vi "Interpret Driver Controls.vi"() -> ()   [LabVIEW 2018]
uses:
  <vilib>/Rock Robotics/WPI/DriverStation/WPI_DriverStationDerivedRobotMode.ctl
  Robot Global Data.vi
  SubSystems/Controllers/Driver Controller/Driver Controller Global.vi
  SubSystems/Lift/Lift Global.vi
  SubSystems/Drive Train/Drive Train Global.vi
  SubSystems/Controllers/Manipulator Controlller/Manipulator Controller Global.vi
  SubSystems/HAB Climber/HAB Climber Global.vi
  SubSystems/Cargo Intake/Cargo Intake Global.vi
  SubSystems/Hatch Panel Intake/Hatch Panel Intake Global.vi
  <vilib>/addons/control/pid/pid.llb/PID (DBL).vi
  <vilib>/addons/control/pid/NI_PID_pid.lvlib
panel:
  in  "Rot. Point Y":dbl
  in  "Rot. Point X":dbl
  in  "robot centric":bool
  in  "Z speed":dbl=1.0
  in  "Y Speed":dbl=1.0
  in  "X Speed":dbl=1.0
  out "Grab Hatch Boolean Thing":bool=TRUE
  in  "Track Scale":dbl
  in  "Last Move Deadband":u32=500
  in  "Last Time Auto":u32=1816077
  in  "Camera Tracking":T1={"proportional gain (Kc)"=0.06, "integral time (Ti, min)"=0.0, "derivative time (Td, min)"=0.0}
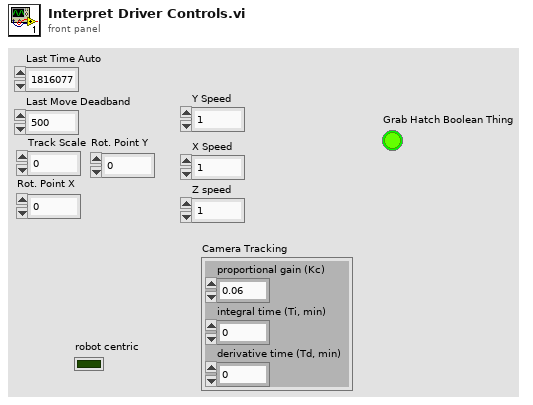
[diagram p1: front panel]
types:
  T1 = cluster{"proportional gain (Kc)":dbl, "integral time (Ti, min)":dbl, "derivative time (Td, min)":dbl}
  T2 = enum16{"Manual", "Hatch Panel Zone 1", "Hatch Panel Zone 2", "Hatch Panel Zone 3", "Cargo Zone 1", "Cargo Zone 2", "Cargo Zone 3", "Cargo Ship Zone"}
  T3 = enum16{"Hatch Panel Zone 1", "Hatch Panel Zone 2", "Hatch Panel Zone 3", "Cargo Zone 1", "Cargo Zone 2", "Cargo Zone 3", "Cargo Ship Zone"}
  T4 = typedef "WPI_DriverStationDerivedRobotMode.ctl" = enum16{"Init", "Execute", "Stop"}
  T5 = cluster{"Rollover":dbl, "Yaw":dbl, "Cont Yaw":dbl}
  T6 = cluster{"offsetAngle H":dbl, "offsetAngle V":dbl, "area":dbl, "skew":dbl, "validTarget":dbl, "latency":dbl}
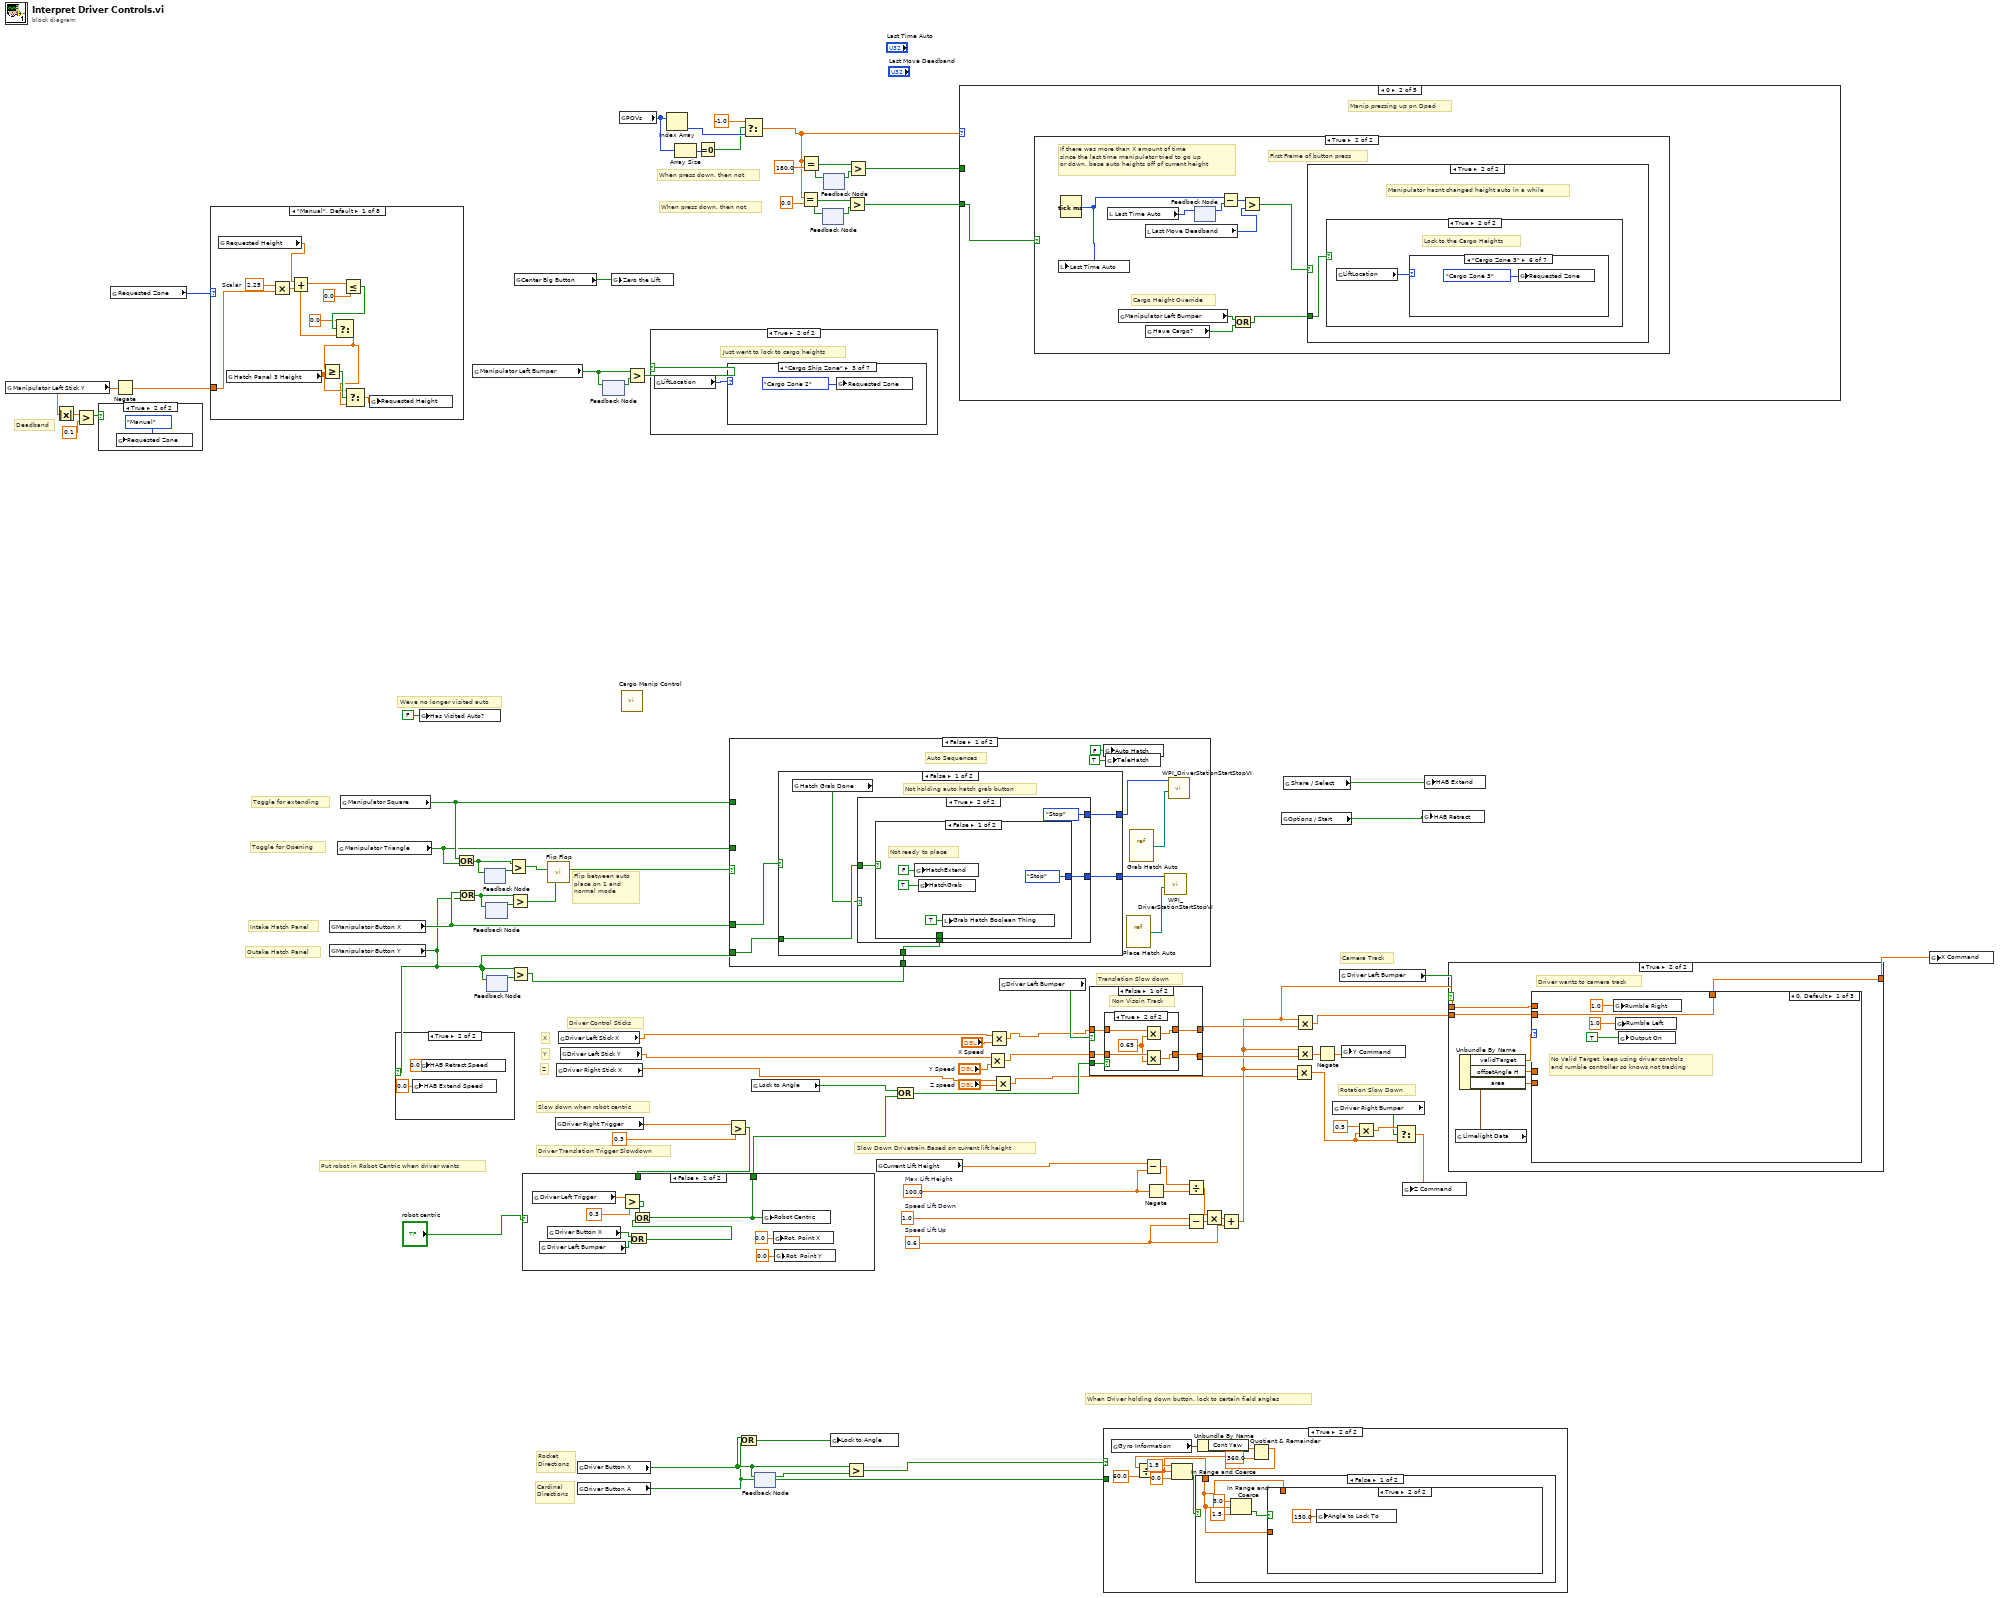
[diagram p0: block diagram]
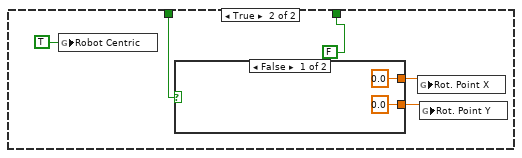
[diagram p3: hidden frame]
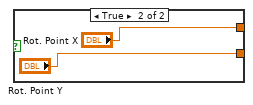
[diagram p4: hidden frame]
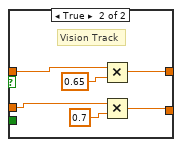
[diagram p6: hidden frame]
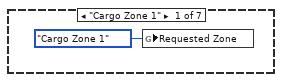
[diagram p8: hidden frame]
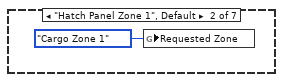
[diagram p9: hidden frame]
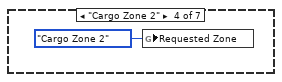
[diagram p10: hidden frame]
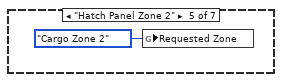
[diagram p11: hidden frame]
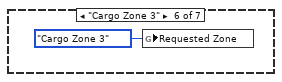
[diagram p12: hidden frame]
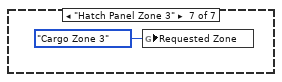
[diagram p13: hidden frame]
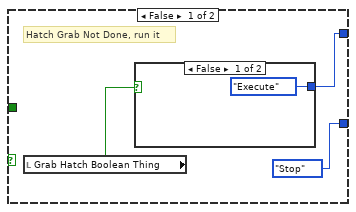
[diagram p14: hidden frame]
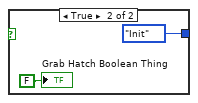
[diagram p15: hidden frame]
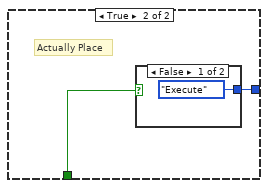
[diagram p16: hidden frame]
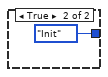
[diagram p17: hidden frame]
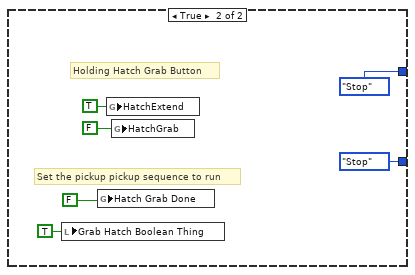
[diagram p18: hidden frame]
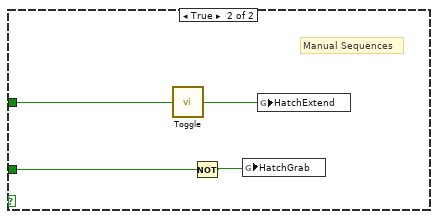
[diagram p19: hidden frame]
diagram:
  w70 = 0.6  # Speed Lift Up
  w74 = 1.0  # Speed Lift Down
  w68 = 100.0  # Max Lift Height
  # "Toggle for Opening"
  # "Toggle for extending"
  # "Outake Hatch Panel"
  # "Intake Hatch Panel"
  # "Flip between auto\nplace on 1 and \nnormal mode"
  # "When press down, then not"
  # "When press down, then not"
  # "Deadband"
  # "Weve no longer visited auto"
  # "Camera Track"
  # "Rotation Slow Down"
  # "Rocket\nDirections"
  # "Cardinal\nDirections"
  # "When Driver holding down button, lock to certain field angles"
  # "Slow Down Drivetrain Based on current lift height"
  # "Put robot in Robot Centric when driver wants"
  # "Slow down when robot centric"
  # "Driver Translation Trigger Slowdown"
  # "Translation Slow down"
  # "Z"
  # "Y"
  # "X"
  # "Driver Control Sticks"
  n1 = global read "Manipulator Controller Global.vi" "Manipulator Left Stick Y"() -> (w44:dbl)
  n2 = Absolute Value(x=w44) -> (abs(x)=w47:dbl)
  n3 = Greater?(x=w47, y=0.1) -> (0:w45:bool)
  n4 = case shown="True" w45 {
    frame False {
    }
    frame True {
      n5 = global write "Lift Global.vi" "Requested Zone"(T2."Manual" ("Requested Zone")) -> ()
    }
  }
  n6 = global read "Lift Global.vi" "Requested Zone"() -> (w48:T2)
  n7 = Negate(x=w44) -> (-x=w43:dbl)
  n8 = case shown="\"Manual\", Default" w48 {
    tunnel: w43 -> [w95 _ _ _ _ _ _ _]
    frame "Manual", Default {
      w94 = 2.25  # Scalar
      n9 = global read "Lift Global.vi" "Requested Height"() -> (w97:dbl)
      n10 = global read "Lift Global.vi" "Hatch Panel 3 Height"() -> (w88:dbl)
      n11 = Multiply(x=w94, y=w95) -> (x*y=w96:dbl)
      n12 = Add(x=w97, y=w96) -> (x+y=w90:dbl)
      n13 = Less Or Equal?(x=w90, y=0.0) -> (x <= y?=w92:bool)
      n14 = Select(t=0.0, s=w92, f=w90) -> (s? t:f=w87:dbl)
      n15 = Greater Or Equal?(x=w87, y=w88) -> (x >= y?=w89:bool)
      n16 = Select(t=w88, s=w89, f=w87) -> (s? t:f=w86:dbl)
      n17 = global write "Lift Global.vi" "Requested Height"(w86) -> ()
    }
    frame "Hatch Panel Zone 1" {
      n18 = global read "Lift Global.vi" "Hatch Panel 1 Height"() -> (w98:dbl)
      n19 = global write "Lift Global.vi" "Requested Height"(w98) -> ()
    }
    frame "Hatch Panel Zone 2" {
      n20 = global read "Lift Global.vi" "Hatch Panel 2 Height"() -> (w99:dbl)
      n21 = global write "Lift Global.vi" "Requested Height"(w99) -> ()
    }
    frame "Hatch Panel Zone 3" {
      n22 = global read "Lift Global.vi" "Hatch Panel 3 Height"() -> (w100:dbl)
      n23 = global write "Lift Global.vi" "Requested Height"(w100) -> ()
    }
    frame "Cargo Zone 1" {
      n24 = global read "Lift Global.vi" "Cargo Zone 1 Height"() -> (w101:dbl)
      n25 = global write "Lift Global.vi" "Requested Height"(w101) -> ()
    }
    frame "Cargo Zone 2" {
      n26 = global read "Lift Global.vi" "Cargo Zone 2 Height"() -> (w102:dbl)
      n27 = global write "Lift Global.vi" "Requested Height"(w102) -> ()
    }
    frame "Cargo Zone 3" {
      n28 = global read "Lift Global.vi" "Cargo Zone 3 Height"() -> (w103:dbl)
      n29 = global write "Lift Global.vi" "Requested Height"(w103) -> ()
    }
    frame "Cargo Ship Zone" {
      n30 = global read "Lift Global.vi" "Cargo Ship Height"() -> (w104:dbl)
      n31 = global write "Lift Global.vi" "Requested Height"(w104) -> ()
    }
  }
  n32 = global read "Manipulator Controller Global.vi" "Manipulator Button X"() -> (w20:bool)
  n33 = global read "Manipulator Controller Global.vi" "Manipulator Button Y"() -> (w4:bool)
  n34 = global read "Manipulator Controller Global.vi" "Manipulator Triangle"() -> (w30:bool)
  n35 = global read "Manipulator Controller Global.vi" "Manipulator Square"() -> (w31:bool)
  n36 = case shown="True" w4 {
    frame False {
    }
    frame True {
      n37 = global write "HAB Climber Global.vi" "HAB Extend Speed"(0.0 ("HAB Extend Speed")) -> ()
      n38 = global write "HAB Climber Global.vi" "HAB Retract Speed"(0.0 ("HAB Retract Speed")) -> ()
    }
  }
  n39 = global write "Robot Global Data.vi" "Has Visited Auto?"(FALSE ("Has Visited Auto?")) -> ()
  n40 = Or(x=w31, y=w30) -> (x .or. y?=w28:bool)
  n41 = Or(x=w20, y=w4) -> (x .or. y?=w25:bool)
  n42 = global read "Manipulator Controller Global.vi" "Manipulator Left Bumper"() -> (w18:bool)
  n43 = feedback-in #1(w28) -> ()
  n44 = feedback #1() -> (w29:bool)  [unwired: 1 in]
  n45 = feedback #2() -> (w26:bool)  [unwired: 1 in]
  n46 = feedback-in #2(w25) -> ()
  n47 = feedback #3() -> (w22:bool)  [unwired: 1 in]
  n48 = feedback-in #3(w4) -> ()
  n49 = Greater?(x=w28, y=w29) -> (0:w27:bool)
  n50 = Greater?(x=w25, y=w26) -> (0:w24:bool)
  n51 = Greater?(x=w4, y=w22) -> (0:w21:bool)
  n52 = global read "Manipulator Controller Global.vi" "Center Big Button"() -> (w14:bool)
  n53 = call "Flip Flop.vi"("Line 2"=w24, "Line 1"=w27) -> ("Switch"=w23:bool)  [unwired: 9 in]
  n54 = global read "Driver Controller Global.vi" "Driver Right Trigger"() -> (w84:dbl)
  n55 = global read "Driver Controller Global.vi" "Driver Right Stick X"() -> (w7:dbl)
  n56 = global read "Driver Controller Global.vi" "Driver Left Stick X"() -> (w16:dbl)
  n57 = global read "Driver Controller Global.vi" "Driver Left Stick Y"() -> (w15:dbl)
  n58 = global read "Driver Controller Global.vi" "Driver Button X"() -> (w66:bool)
  n59 = global read "Driver Controller Global.vi" "Driver Button A"() -> (w64:bool)
  n60 = feedback #4() -> (w19:bool)  [unwired: 1 in]
  n61 = feedback-in #4(w18) -> ()
  n62 = global write "Lift Global.vi" "Zero the Lift"(w14) -> ()
  n63 = global read "Manipulator Controller Global.vi" "POVs"() -> (w52:i16[])
  n64 = call "Cargo Manip Control.vi"() -> ()  [unwired: 12 in]
  n65 = Greater?(x=w18, y=w19) -> (0:w17:bool)
  n66 = case shown="True" w17 {
    frame False {
    }
    frame True {
      # "Just went to lock to cargo heights"
      n67 = global read "Lift Global.vi" "LiftLocation"() -> (w107:T3)
      n68 = case shown="\"Cargo Ship Zone\"" w107 {
        frame "Cargo Zone 1" {
          n69 = global write "Lift Global.vi" "Requested Zone"(T2."Cargo Zone 1" ("Requested Zone")) -> ()
        }
        frame "Hatch Panel Zone 1", Default {
          n70 = global write "Lift Global.vi" "Requested Zone"(T2."Cargo Zone 1" ("Requested Zone")) -> ()
        }
        frame "Cargo Ship Zone" {
          n71 = global write "Lift Global.vi" "Requested Zone"(T2."Cargo Zone 2" ("Requested Zone")) -> ()
        }
        frame "Cargo Zone 2" {
          n72 = global write "Lift Global.vi" "Requested Zone"(T2."Cargo Zone 2" ("Requested Zone")) -> ()
        }
        frame "Hatch Panel Zone 2" {
          n73 = global write "Lift Global.vi" "Requested Zone"(T2."Cargo Zone 2" ("Requested Zone")) -> ()
        }
        frame "Cargo Zone 3" {
          n74 = global write "Lift Global.vi" "Requested Zone"(T2."Cargo Zone 3" ("Requested Zone")) -> ()
        }
        frame "Hatch Panel Zone 3" {
          n75 = global write "Lift Global.vi" "Requested Zone"(T2."Cargo Zone 3" ("Requested Zone")) -> ()
        }
      }
    }
  }
  n76 = Index Array(array=w52) -> (element=w49:i16)  [unwired: 1 in]
  n77 = Array Size(array=w52) -> (size(s)=w51:i32)
  n78 = Equal To 0?(x=w51) -> (x = 0?=w42:bool)
  n79 = Greater?(x=w84, y=0.3) -> (0:w5:bool)
  n80 = case shown="False" "robot centric" {
    tunnel: [w117 FALSE] -> w12
    tunnel: w5 -> [_ w126]
    frame False {
      n81 = global read "Driver Controller Global.vi" "Driver Left Trigger"() -> (w122:dbl)
      n82 = global read "Driver Controller Global.vi" "Driver Left Bumper"() -> (w118:bool)
      n83 = global read "Driver Controller Global.vi" "Driver Button X"() -> (w119:bool)
      n84 = Greater?(x=w122, y=0.3) -> (0:w121:bool)
      n85 = Or(x=w119, y=w118) -> (x .or. y?=w120:bool)
      n86 = Or(x=w121, y=w120) -> (x .or. y?=w117:bool)
      n87 = global write "Drive Train Global.vi" "Robot Centric"(w117) -> ()
      n88 = global write "Drive Train Global.vi" "Rot. Point X"(0.0 ("Rot. Point X")) -> ()
      n89 = global write "Drive Train Global.vi" "Rot. Point Y"(0.0 ("Rot. Point Y")) -> ()
    }
    frame True {
      n90 = global write "Drive Train Global.vi" "Robot Centric"(TRUE ("Robot Centric")) -> ()
      n91 = case shown="False" w126 {
        tunnel: [0.0 ("Rot. Point Y") "Rot. Point Y"] -> w125
        tunnel: [0.0 ("Rot. Point X") "Rot. Point X"] -> w124
        frame False {
        }
        frame True {
        }
      }
      n92 = global write "Drive Train Global.vi" "Rot. Point X"(w124) -> ()
      n93 = global write "Drive Train Global.vi" "Rot. Point Y"(w125) -> ()
    }
  }
  n94 = case shown="False" w23 {
    tunnel: w30 -> [_ w172]
    tunnel: w31 -> [_ w173]
    tunnel: w20 -> [w141 _]
    tunnel: w21 -> [w138 _]
    tunnel: w4 -> [w137 _]
    frame False {
      # "Auto Sequences"
      n95 = case shown="False" w141 {
        tunnel: [w146 WPI_DriverStationDerivedRobotMode."Stop" ("Call Context")] -> w139
        tunnel: w138 -> [w145 _]
        tunnel: w137 -> [w144 _]
        tunnel: [w142 WPI_DriverStationDerivedRobotMode."Stop" ("Call Context")] -> w135
        frame False {
          # "Not holding auto hatch grab button"
          n96 = global read "Hatch Panel Intake Global.vi" "Hatch Grab Done"() -> (w143:bool)
          n97 = case shown="True" w143 {
            tunnel: [WPI_DriverStationDerivedRobotMode."Stop" ("Call Context") w156] -> w146
            tunnel: w145 -> [_ w155]
            tunnel: w144 -> [_ w154]
            tunnel: [w149 WPI_DriverStationDerivedRobotMode."Stop" ("Call Context")] -> w142
            frame False {
              # "Hatch Grab Not Done, run it"
              n98 = local read "Grab Hatch Boolean Thing"() -> (w147:bool)
              n99 = case shown="False" w147 {
                tunnel: [WPI_DriverStationDerivedRobotMode."Execute" ("Call Context") WPI_DriverStationDerivedRobotMode."Init" ("Call Context")] -> w149
                frame False {
                }
                frame True {
                  "Grab Hatch Boolean Thing" <- FALSE ("Grab Hatch Boolean Thing")
                }
              }
            }
            frame True {
              n100 = case shown="False" w154 {
                tunnel: [WPI_DriverStationDerivedRobotMode."Stop" ("Call Context") w162] -> w156
                tunnel: w155 -> [_ w161]
                frame False {
                  # "Not ready to place"
                  n101 = global write "Hatch Panel Intake Global.vi" "HatchExtend"(FALSE ("HatchExtend")) -> ()
                  n102 = global write "Hatch Panel Intake Global.vi" "HatchGrab"(TRUE ("HatchExtend")) -> ()
                  n103 = local write "Grab Hatch Boolean Thing"(TRUE ("Grab Hatch Boolean Thing")) -> ()
                }
                frame True {
                  # "Actually Place"
                  n104 = case shown="False" w161 {
                    tunnel: [WPI_DriverStationDerivedRobotMode."Execute" ("Call Context") WPI_DriverStationDerivedRobotMode."Init" ("Call Context")] -> w162
                    frame False {
                    }
                    frame True {
                    }
                  }
                }
              }
            }
          }
        }
        frame True {
          # "Set the pickup pickup sequence to run"
          # "Holding Hatch Grab Button"
          n105 = local write "Grab Hatch Boolean Thing"(TRUE ("Grab Hatch Boolean Thing")) -> ()
          n106 = global write "Hatch Panel Intake Global.vi" "Hatch Grab Done"(FALSE ("HatchExtend")) -> ()
          n107 = global write "Hatch Panel Intake Global.vi" "HatchExtend"(TRUE ("HatchExtend")) -> ()
          n108 = global write "Hatch Panel Intake Global.vi" "HatchGrab"(FALSE ("HatchExtend")) -> ()
        }
      }
      n109 = global write "Hatch Panel Intake Global.vi" "Auto Hatch"(FALSE ("TeleHatch")) -> ()
      n110 = global write "Hatch Panel Intake Global.vi" "TeleHatch"(TRUE ("TeleHatch")) -> ()
      n111 = vi-ref "Place Hatch Auto.vi"() -> (w140:refnum<vi>)
      n112 = vi-ref "Grab Hatch Auto.vi"() -> (w136:refnum<vi>)
      n113 = call <vilib>:"WPI_DriverStationStartStopVI.vi"("VI in"=w140, "Call Context"=w139) -> ()  [unwired: 10 in]
      n114 = call <vilib>:"WPI_DriverStationStartStopVI.vi"("VI in"=w136, "Call Context"=w135) -> ()  [unwired: 10 in]
    }
    frame True {
      # "Manual Sequences"
      n115 = call "Toggle.vi"("Input"=w173) -> ("Output"=w174:bool)
      n116 = Not(x=w172) -> (.not. x?=w171:bool)
      n117 = global write "Hatch Panel Intake Global.vi" "HatchGrab"(w171) -> ()
      n118 = global write "Hatch Panel Intake Global.vi" "HatchExtend"(w174) -> ()
    }
  }
  n119 = Or(x=w66, y=w64) -> (x .or. y?=w63:bool)
  n120 = Select(t=-1.0, s=w42, f=w49) -> (s? t:f=w34:dbl)
  n121 = global read "Drive Train Global.vi" "Lock to Angle"() -> (w62:bool)
  n122 = feedback #5() -> (w67:bool)  [unwired: 1 in]
  n123 = feedback-in #5(w66) -> ()
  n124 = Equal?(x=w34, y=0.0) -> (x = y?=w37:bool)
  n125 = Equal?(x=w34, y=180.0) -> (x = y?=w39:bool)
  n126 = feedback #6() -> (w36:bool)  [unwired: 1 in]
  n127 = feedback-in #6(w37) -> ()
  n128 = feedback-in #7(w39) -> ()
  n129 = feedback #7() -> (w40:bool)  [unwired: 1 in]
  n130 = global write "Drive Train Global.vi" "Lock to Angle"(w63) -> ()
  n131 = Greater?(x=w66, y=w67) -> (0:w65:bool)
  n132 = Greater?(x=w37, y=w36) -> (0:w33:bool)
  n133 = Greater?(x=w39, y=w40) -> (0:w38:bool)
  n134 = global read "Lift Global.vi" "Current Lift Height"() -> (w76:dbl)
  n135 = Compound Arithmetic op=OR(w62, w12) -> (w9:bool)
  n136 = case shown="0" w34 {
    tunnel: w38 -> [_ _ w219 _ _]
    tunnel: w33 -> [_ w175 _ _ _]
    frame -1, Default {
      # "Nothing on the D-Pad is pressed!"
    }
    frame 0 {
      # "Manip pressing up on Dpad"
      n137 = case shown="True" w175 {
        frame False {
          # "Still pressing button, do nothing"
        }
        frame True {
          # "Cargo Height Override"
          # "First Frame of button press"
          # "If there was more than X amount of time\nsince the last time manipulator tried to go up\nor down, base auto heights off of current height"
          n138 = Tick Count (ms)() -> (millisecond timer value=w181:u32)
          n139 = local write "Last Time Auto"(w181) -> ()
          n140 = local read "Last Time Auto"() -> (w180:u32)
          n141 = global read "Manipulator Controller Global.vi" "Manipulator Left Bumper"() -> (w178:bool)
          n142 = local read "Last Move Deadband"() -> (w182:u32)
          n143 = global read "Cargo Intake Global.vi" "Have Cargo?"() -> (w176:bool)
          n144 = feedback #8() -> (w179:u32)  [unwired: 1 in]
          n145 = feedback-in #8(w180) -> ()
          n146 = Subtract(x=w181, y=w179) -> (x-y=w184:u32)
          n147 = Or(x=w178, y=w176) -> (x .or. y?=w177:bool)
          n148 = Greater?(x=w184, y=w182) -> (0:w183:bool)
          n149 = case shown="True" w183 {
            tunnel: w177 -> [w185 w202]
            frame False {
              # "Manipulator is still changing height to go to"
              n150 = case shown="False" w185 {
                frame False {
                  # "Lock to the Hatch Heights"
                  n151 = global read "Lift Global.vi" "Requested Zone"() -> (w186:T2)
                  n152 = case shown="\"Hatch Panel Zone 3\"" w186 {
                    frame "Manual" {
                    }
                    frame "Cargo Zone 1" {
                      n153 = global write "Lift Global.vi" "Requested Zone"(T2."Hatch Panel Zone 1" ("Requested Zone")) -> ()
                    }
                    frame "Hatch Panel Zone 1", Default {
                      n154 = global write "Lift Global.vi" "Requested Zone"(T2."Hatch Panel Zone 2" ("Requested Zone")) -> ()
                    }
                    frame "Cargo Ship Zone" {
                      n155 = global write "Lift Global.vi" "Requested Zone"(T2."Hatch Panel Zone 2" ("Requested Zone")) -> ()
                    }
                    frame "Cargo Zone 2" {
                      n156 = global write "Lift Global.vi" "Requested Zone"(T2."Hatch Panel Zone 2" ("Requested Zone")) -> ()
                    }
                    frame "Hatch Panel Zone 2" {
                      n157 = global write "Lift Global.vi" "Requested Zone"(T2."Hatch Panel Zone 3" ("Requested Zone")) -> ()
                    }
                    frame "Cargo Zone 3" {
                      n158 = global write "Lift Global.vi" "Requested Zone"(T2."Hatch Panel Zone 3" ("Requested Zone")) -> ()
                    }
                    frame "Hatch Panel Zone 3" {
                      n159 = global write "Lift Global.vi" "Requested Zone"(T2."Hatch Panel Zone 3" ("Requested Zone")) -> ()
                    }
                  }
                }
                frame True {
                  # "Lock to the Cargo Heights"
                  n160 = global read "Lift Global.vi" "Requested Zone"() -> (w194:T2)
                  n161 = case shown="\"Manual\"" w194 {
                    frame "Manual" {
                    }
                    frame "Cargo Zone 1" {
                      n162 = global write "Lift Global.vi" "Requested Zone"(T2."Cargo Zone 2" ("Requested Zone")) -> ()
                    }
                    frame "Hatch Panel Zone 1", Default {
                      n163 = global write "Lift Global.vi" "Requested Zone"(T2."Cargo Zone 2" ("Requested Zone")) -> ()
                    }
                    frame "Cargo Ship Zone" {
                      n164 = global write "Lift Global.vi" "Requested Zone"(T2."Cargo Zone 2" ("Requested Zone")) -> ()
                    }
                    frame "Cargo Zone 2" {
                      n165 = global write "Lift Global.vi" "Requested Zone"(T2."Cargo Zone 3" ("Requested Zone")) -> ()
                    }
                    frame "Hatch Panel Zone 2" {
                      n166 = global write "Lift Global.vi" "Requested Zone"(T2."Cargo Zone 3" ("Requested Zone")) -> ()
                    }
                    frame "Cargo Zone 3" {
                      n167 = global write "Lift Global.vi" "Requested Zone"(T2."Cargo Zone 3" ("Requested Zone")) -> ()
                    }
                    frame "Hatch Panel Zone 3" {
                      n168 = global write "Lift Global.vi" "Requested Zone"(T2."Cargo Zone 3" ("Requested Zone")) -> ()
                    }
                  }
                }
              }
            }
            frame True {
              # "Manipulator hasnt changed height auto in a while"
              n169 = case shown="True" w202 {
                frame False {
                  # "Lock to the Hatch Heights"
                  n170 = global read "Lift Global.vi" "LiftLocation"() -> (w203:T3)
                  n171 = case shown="\"Cargo Zone 1\"" w203 {
                    frame "Cargo Zone 1" {
                      n172 = global write "Lift Global.vi" "Requested Zone"(T2."Hatch Panel Zone 1" ("Requested Zone")) -> ()
                    }
                    frame "Hatch Panel Zone 1", Default {
                      n173 = global write "Lift Global.vi" "Requested Zone"(T2."Hatch Panel Zone 2" ("Requested Zone")) -> ()
                    }
                    frame "Cargo Ship Zone" {
                      n174 = global write "Lift Global.vi" "Requested Zone"(T2."Hatch Panel Zone 2" ("Requested Zone")) -> ()
                    }
                    frame "Cargo Zone 2" {
                      n175 = global write "Lift Global.vi" "Requested Zone"(T2."Hatch Panel Zone 2" ("Requested Zone")) -> ()
                    }
                    frame "Hatch Panel Zone 2" {
                      n176 = global write "Lift Global.vi" "Requested Zone"(T2."Hatch Panel Zone 3" ("Requested Zone")) -> ()
                    }
                    frame "Cargo Zone 3" {
                      n177 = global write "Lift Global.vi" "Requested Zone"(T2."Hatch Panel Zone 3" ("Requested Zone")) -> ()
                    }
                    frame "Hatch Panel Zone 3" {
                      n178 = global write "Lift Global.vi" "Requested Zone"(T2."Hatch Panel Zone 3" ("Requested Zone")) -> ()
                    }
                  }
                }
                frame True {
                  # "Lock to the Cargo Heights"
                  n179 = global read "Lift Global.vi" "LiftLocation"() -> (w211:T3)
                  n180 = case shown="\"Cargo Zone 3\"" w211 {
                    frame "Cargo Zone 1" {
                      n181 = global write "Lift Global.vi" "Requested Zone"(T2."Cargo Zone 2" ("Requested Zone")) -> ()
                    }
                    frame "Hatch Panel Zone 1", Default {
                      n182 = global write "Lift Global.vi" "Requested Zone"(T2."Cargo Zone 2" ("Requested Zone")) -> ()
                    }
                    frame "Cargo Ship Zone" {
                      n183 = global write "Lift Global.vi" "Requested Zone"(T2."Cargo Zone 2" ("Requested Zone")) -> ()
                    }
                    frame "Cargo Zone 2" {
                      n184 = global write "Lift Global.vi" "Requested Zone"(T2."Cargo Zone 3" ("Requested Zone")) -> ()
                    }
                    frame "Hatch Panel Zone 2" {
                      n185 = global write "Lift Global.vi" "Requested Zone"(T2."Cargo Zone 3" ("Requested Zone")) -> ()
                    }
                    frame "Cargo Zone 3" {
                      n186 = global write "Lift Global.vi" "Requested Zone"(T2."Cargo Zone 3" ("Requested Zone")) -> ()
                    }
                    frame "Hatch Panel Zone 3" {
                      n187 = global write "Lift Global.vi" "Requested Zone"(T2."Cargo Zone 3" ("Requested Zone")) -> ()
                    }
                  }
                }
              }
            }
          }
        }
      }
    }
    frame 180 {
      # "Manip pressing down on Dpad"
      n188 = case shown="True" w219 {
        frame False {
          # "Still pressing button, do nothing"
        }
        frame True {
          # "Cargo Height Override"
          # "First frame of button press"
          # "If there was more than X amount of time\nsince the last time manipulator tried to go up\nor down, base auto heights off of current height"
          n189 = Tick Count (ms)() -> (millisecond timer value=w227:u32)
          n190 = local write "Last Time Auto"(w227) -> ()
          n191 = local read "Last Time Auto"() -> (w225:u32)
          n192 = global read "Manipulator Controller Global.vi" "Manipulator Left Bumper"() -> (w222:bool)
          n193 = local read "Last Move Deadband"() -> (w226:u32)
          n194 = global read "Cargo Intake Global.vi" "Have Cargo?"() -> (w221:bool)
          n195 = feedback #9() -> (w224:u32)  [unwired: 1 in]
          n196 = feedback-in #9(w225) -> ()
          n197 = Subtract(x=w227, y=w224) -> (x-y=w228:u32)
          n198 = Greater?(x=w228, y=w226) -> (0:w223:bool)
          n199 = Or(x=w222, y=w221) -> (x .or. y?=w220:bool)
          n200 = case shown="False" w223 {
            tunnel: w220 -> [w229 w246]
            frame False {
              # "Manipulator is still changing height to go to"
              n201 = case shown="False" w229 {
                frame False {
                  # "Lock to the Hatch Heights"
                  n202 = global read "Lift Global.vi" "Requested Zone"() -> (w230:T2)
                  n203 = case shown="\"Hatch Panel Zone 3\"" w230 {
                    frame "Manual" {
                    }
                    frame "Cargo Zone 1" {
                      n204 = global write "Lift Global.vi" "Requested Zone"(T2."Hatch Panel Zone 1" ("Requested Zone")) -> ()
                    }
                    frame "Hatch Panel Zone 1", Default {
                      n205 = global write "Lift Global.vi" "Requested Zone"(T2."Hatch Panel Zone 1" ("Requested Zone")) -> ()
                    }
                    frame "Cargo Ship Zone" {
                      n206 = global write "Lift Global.vi" "Requested Zone"(T2."Hatch Panel Zone 1" ("Requested Zone")) -> ()
                    }
                    frame "Cargo Zone 2" {
                      n207 = global write "Lift Global.vi" "Requested Zone"(T2."Hatch Panel Zone 1" ("Requested Zone")) -> ()
                    }
                    frame "Hatch Panel Zone 2" {
                      n208 = global write "Lift Global.vi" "Requested Zone"(T2."Hatch Panel Zone 1" ("Requested Zone")) -> ()
                    }
                    frame "Cargo Zone 3" {
                      n209 = global write "Lift Global.vi" "Requested Zone"(T2."Hatch Panel Zone 2" ("Requested Zone")) -> ()
                    }
                    frame "Hatch Panel Zone 3" {
                      n210 = global write "Lift Global.vi" "Requested Zone"(T2."Hatch Panel Zone 2" ("Requested Zone")) -> ()
                    }
                  }
                }
                frame True {
                  # "Lock to the Cargo Heights"
                  n211 = global read "Lift Global.vi" "Requested Zone"() -> (w238:T2)
                  n212 = case shown="\"Manual\"" w238 {
                    frame "Manual" {
                    }
                    frame "Cargo Zone 1" {
                      n213 = global write "Lift Global.vi" "Requested Zone"(T2."Cargo Zone 1" ("Requested Zone")) -> ()
                    }
                    frame "Hatch Panel Zone 1", Default {
                      n214 = global write "Lift Global.vi" "Requested Zone"(T2."Cargo Zone 1" ("Requested Zone")) -> ()
                    }
                    frame "Cargo Ship Zone" {
                      n215 = global write "Lift Global.vi" "Requested Zone"(T2."Cargo Zone 1" ("Requested Zone")) -> ()
                    }
                    frame "Cargo Zone 2" {
                      n216 = global write "Lift Global.vi" "Requested Zone"(T2."Cargo Zone 1" ("Requested Zone")) -> ()
                    }
                    frame "Hatch Panel Zone 2" {
                      n217 = global write "Lift Global.vi" "Requested Zone"(T2."Cargo Zone 2" ("Requested Zone")) -> ()
                    }
                    frame "Cargo Zone 3" {
                      n218 = global write "Lift Global.vi" "Requested Zone"(T2."Cargo Zone 2" ("Requested Zone")) -> ()
                    }
                    frame "Hatch Panel Zone 3" {
                      n219 = global write "Lift Global.vi" "Requested Zone"(T2."Cargo Zone 3" ("Requested Zone")) -> ()
                    }
                  }
                }
              }
            }
            frame True {
              # "Manipulator hasnt changed height auto in a while"
              n220 = case shown="False" w246 {
                frame False {
                  # "Lock to the Hatch Heights"
                  n221 = global read "Lift Global.vi" "LiftLocation"() -> (w247:T3)
                  n222 = case shown="\"Hatch Panel Zone 3\"" w247 {
                    frame "Cargo Zone 1" {
                      n223 = global write "Lift Global.vi" "Requested Zone"(T2."Hatch Panel Zone 1" ("Requested Zone")) -> ()
                    }
                    frame "Hatch Panel Zone 1", Default {
                      n224 = global write "Lift Global.vi" "Requested Zone"(T2."Hatch Panel Zone 1" ("Requested Zone")) -> ()
                    }
                    frame "Cargo Ship Zone" {
                      n225 = global write "Lift Global.vi" "Requested Zone"(T2."Hatch Panel Zone 1" ("Requested Zone")) -> ()
                    }
                    frame "Cargo Zone 2" {
                      n226 = global write "Lift Global.vi" "Requested Zone"(T2."Hatch Panel Zone 1" ("Requested Zone")) -> ()
                    }
                    frame "Hatch Panel Zone 2" {
                      n227 = global write "Lift Global.vi" "Requested Zone"(T2."Hatch Panel Zone 1" ("Requested Zone")) -> ()
                    }
                    frame "Cargo Zone 3" {
                      n228 = global write "Lift Global.vi" "Requested Zone"(T2."Hatch Panel Zone 2" ("Requested Zone")) -> ()
                    }
                    frame "Hatch Panel Zone 3" {
                      n229 = global write "Lift Global.vi" "Requested Zone"(T2."Hatch Panel Zone 2" ("Requested Zone")) -> ()
                    }
                  }
                }
                frame True {
                  # "Lock to the Cargo Heights"
                  n230 = global read "Lift Global.vi" "LiftLocation"() -> (w255:T3)
                  n231 = case shown="\"Hatch Panel Zone 3\"" w255 {
                    frame "Cargo Zone 1" {
                      n232 = global write "Lift Global.vi" "Requested Zone"(T2."Cargo Zone 1" ("Requested Zone")) -> ()
                    }
                    frame "Hatch Panel Zone 1", Default {
                      n233 = global write "Lift Global.vi" "Requested Zone"(T2."Cargo Zone 1" ("Requested Zone")) -> ()
                    }
                    frame "Cargo Ship Zone" {
                      n234 = global write "Lift Global.vi" "Requested Zone"(T2."Cargo Zone 1" ("Requested Zone")) -> ()
                    }
                    frame "Cargo Zone 2" {
                      n235 = global write "Lift Global.vi" "Requested Zone"(T2."Cargo Zone 1" ("Requested Zone")) -> ()
                    }
                    frame "Hatch Panel Zone 2" {
                      n236 = global write "Lift Global.vi" "Requested Zone"(T2."Cargo Zone 2" ("Requested Zone")) -> ()
                    }
                    frame "Cargo Zone 3" {
                      n237 = global write "Lift Global.vi" "Requested Zone"(T2."Cargo Zone 2" ("Requested Zone")) -> ()
                    }
                    frame "Hatch Panel Zone 3" {
                      n238 = global write "Lift Global.vi" "Requested Zone"(T2."Cargo Zone 3" ("Requested Zone")) -> ()
                    }
                  }
                }
              }
            }
          }
        }
      }
    }
    frame 90 {
      # "Go to Cargo in Cargo Ship Height"
      # "Right on D-Pad"
      n239 = global write "Lift Global.vi" "Requested Zone"(T2."Cargo Ship Zone" ("Requested Zone")) -> ()
    }
    frame 270 {
      # "Go to Hatch Level 1 Height"
      # "Left on D-Pad"
      n240 = global write "Lift Global.vi" "Requested Zone"(T2."Hatch Panel Zone 1" ("Requested Zone")) -> ()
    }
  }
  n241 = Multiply(x=w15, y="Y Speed") -> (x*y=w10:dbl)
  n242 = Multiply(x=w16, y="X Speed") -> (x*y=w11:dbl)
  n243 = Multiply(x=w7, y="Z speed") -> (x*y=w8:dbl)
  n244 = global read "Driver Controller Global.vi" "Driver Left Bumper"() -> (w13:bool)
  n245 = case shown="False" w13 {
    tunnel: w9 -> [w269 _]
    tunnel: [w268 w281] -> w78
    tunnel: [w267 w282] -> w77
    tunnel: w11 -> [w266 w279]
    tunnel: w10 -> [w265 w280]
    frame False {
      # "Non Visoin Track"
      n246 = case shown="True" w269 {
        tunnel: w265 -> [w271 w276]
        tunnel: [w271 w275] -> w268
        tunnel: [w270 w274] -> w267
        tunnel: w266 -> [w270 w273]
        frame False {
        }
        frame True {
          w272 = 0.65 ("Y Slower")
          n247 = Multiply(x=w273, y=w272) -> (x*y=w274:dbl)
          n248 = Multiply(x=w276, y=w272) -> (x*y=w275:dbl)
        }
      }
    }
    frame True {
      # "Vision Track"
      n249 = Multiply(x=w279, y=0.65 ("Y Slower")) -> (x*y=w282:dbl)
      n250 = Multiply(x=w280, y=0.7 ("Y Slower")) -> (x*y=w281:dbl)
    }
  }
  n251 = case shown="True" w65 {
    tunnel: w64 -> [w284 _]
    frame False {
      n252 = feedback #10() -> (w285:bool)  [unwired: 1 in]
      n253 = feedback-in #10(w284) -> ()
      n254 = Greater?(x=w284, y=w285) -> (0:w283:bool)
      n255 = case shown="True" w283 {
        frame False {
        }
        frame True {
          n256 = global read "Drive Train Global.vi" "Gyro Information"() -> (w292:T5)
          n257 = Unbundle By Name(w292) -> ("Yaw"=w289:dbl)
          n258 = Add(x=w289, y=180.0) -> (x+y=w288:dbl)
          n259 = Divide(x=w288, y=90.0) -> (x/y=w290:dbl)
          n260 = Round To Nearest(number=w290) -> (nearest integer value=w286:dbl)
          n261 = case shown="1" w286 {
            frame 0, Default {
              n262 = global write "Drive Train Global.vi" "Angle to Lock To"(180.0 ("Angle to Lock To")) -> ()
            }
            frame 1 {
              n263 = global write "Drive Train Global.vi" "Angle to Lock To"(270.0 ("Angle to Lock To")) -> ()
            }
            frame 2 {
              n264 = global write "Drive Train Global.vi" "Angle to Lock To"(0.0 ("Angle to Lock To")) -> ()
            }
            frame 3 {
              n265 = global write "Drive Train Global.vi" "Angle to Lock To"(90.0 ("Angle to Lock To")) -> ()
            }
            frame 4 {
              n266 = global write "Drive Train Global.vi" "Angle to Lock To"(180.0 ("Angle to Lock To")) -> ()
            }
          }
        }
      }
    }
    frame True {
      n267 = global read "Drive Train Global.vi" "Gyro Information"() -> (w306:T5)
      n268 = Unbundle By Name(w306) -> ("Cont Yaw"=w304:dbl)
      n269 = Quotient & Remainder(x=w304, y=360.0) -> (x-y*floor(x/y)=w302:dbl)  [unwired: 1 out]
      n270 = Divide(x=w302, y=60.0) -> (x/y=w298:dbl)
      n271 = In Range and Coerce(upper limit=1.5, x=w298, lower limit=0.0) -> (In Range?=w299:bool)  [unwired: 1 out]
      n272 = case shown="False" w299 {
        tunnel: w298 -> [w307 _]
        frame False {
          n273 = In Range and Coerce(upper limit=3.0, x=w307, lower limit=1.5) -> (In Range?=w308:bool)  [unwired: 1 out]
          n274 = case shown="True" w308 {
            tunnel: w307 -> [w313 _]
            tunnel: w307 -> [w311 _]
            frame False {
              n275 = In Range and Coerce(upper limit=4.5, x=w313, lower limit=3.0) -> (In Range?=w312:bool)  [unwired: 1 out]
              n276 = case shown="False" w312 {
                tunnel: w311 -> [w317 _]
                frame False {
                  n277 = In Range and Coerce(upper limit=6.0, x=w317, lower limit=4.5) -> (In Range?=w316:bool)  [unwired: 1 out]
                  n278 = case shown="True" w316 {
                    frame False {
                    }
                    frame True {
                      n279 = global write "Drive Train Global.vi" "Angle to Lock To"(330.0 ("Angle to Lock To")) -> ()
                    }
                  }
                }
                frame True {
                  n280 = global write "Drive Train Global.vi" "Angle to Lock To"(210.0 ("Angle to Lock To")) -> ()
                }
              }
            }
            frame True {
              n281 = global write "Drive Train Global.vi" "Angle to Lock To"(150.0 ("Angle to Lock To")) -> ()
            }
          }
        }
        frame True {
          n282 = global write "Drive Train Global.vi" "Angle to Lock To"(30.0 ("Angle to Lock To")) -> ()
        }
      }
    }
  }
  n283 = Subtract(x=w76, y=w68) -> (x-y=w75:dbl)
  n284 = Negate(x=w68) -> (-x=w69:dbl)
  n285 = Divide(x=w75, y=w69) -> (x/y=w73:dbl)
  n286 = Subtract(x=w74, y=w70) -> (x-y=w72:dbl)
  n287 = Multiply(x=w73, y=w72) -> (x*y=w71:dbl)
  n288 = Add(x=w71, y=w70) -> (x+y=w32:dbl)
  n289 = global read "Manipulator Controller Global.vi" "Options / Start"() -> (w56:bool)
  n290 = global read "Manipulator Controller Global.vi" "Share / Select"() -> (w57:bool)
  n291 = Multiply(x=w32, y=w8) -> (x*y=w82:dbl)
  n292 = Multiply(x=w32, y=w77) -> (x*y=w59:dbl)
  n293 = Multiply(x=w32, y=w78) -> (x*y=w55:dbl)
  n294 = Negate(x=w55) -> (-x=w54:dbl)
  n295 = global read "Driver Controller Global.vi" "Driver Right Bumper"() -> (w79:bool)
  n296 = global read "Driver Controller Global.vi" "Driver Left Bumper"() -> (w61:bool)
  n297 = global write "Drive Train Global.vi" "Y Command"(w54) -> ()
  n298 = Multiply(x=0.5, y=w82) -> (x*y=w81:dbl)
  n299 = Select(t=w81, s=w79, f=w82) -> (s? t:f=w60:dbl)
  n300 = global write "Drive Train Global.vi" "Z Command"(w60) -> ()
  n301 = global write "HAB Climber Global.vi" "HAB Retract"(w56) -> ()
  n302 = global write "HAB Climber Global.vi" "HAB Extend"(w57) -> ()
  n303 = case shown="True" w61 {
    tunnel: w59 -> [w325 w330]
    tunnel: [w325 w328] -> w58
    tunnel: w32 -> [_ w327]
    frame False {
      # "Driver not attepting to camera track, be normal"
      n304 = global write "Driver Controller Global.vi" "Output On"(FALSE ("Rumble Controller?")) -> ()
    }
    frame True {
      # "Driver wants to camera track"
      n305 = global read "Robot Global Data.vi" "Limelight Data"() -> (w332:T6)
      n306 = Unbundle By Name(w332) -> ("validTarget"=w331:dbl, "offsetAngle H"=w329:dbl, "area"=w326:dbl)
      n307 = case shown="0, Default" w331 {
        tunnel: w330 -> [w335 _ _]
        tunnel: w329 -> [_ w354 w358]
        tunnel: [w335 w353 w359] -> w328
        tunnel: w327 -> [_ w351 _]
        tunnel: w326 -> [_ w346 _]
        frame 0, Default {
          # "No Valid Target, keep using driver controls\nand rumble controller so knows not tracking"
          n308 = global write "Driver Controller Global.vi" "Rumble Right"(1.0 ("Rumble Amount")) -> ()
          n309 = global write "Driver Controller Global.vi" "Rumble Left"(1.0 ("Rumble Amount")) -> ()
          n310 = global write "Driver Controller Global.vi" "Output On"(TRUE ("Rumble Controller?")) -> ()
        }
        frame 1 {
          # "There is a valid target, track target"
          n311 = Reciprocal(x=w346) -> (1/x=w345:dbl)
          n312 = Unbundle By Name("Camera Tracking") -> ("proportional gain (Kc)"=w339:dbl, "integral time (Ti, min)"=w349:dbl, "derivative time (Td, min)"=w348:dbl)
          n313 = Multiply(x=w345, y="Track Scale") -> (x*y=w338:dbl)
          n314 = Subtract(x=1.0, y="Track Scale") -> (x-y=w342:dbl)
          n315 = Multiply(x=w338, y=w339) -> (x*y=w337:dbl)
          n316 = Multiply(x=w339, y=w342) -> (x*y=w341:dbl)
          n317 = Add(x=w337, y=w341) -> (x+y=w340:dbl)
          n318 = Bundle By Name(cluster="Camera Tracking", "proportional gain (Kc)"=w340, "integral time (Ti, min)"=w349, "derivative time (Td, min)"=w348) -> (w347:T1)
          n319 = call-poly <vilib>:"PID.vi"("output range"=cluster{"output high":dbl, "output low":dbl} {"output high"=1.0, "output low"=-1.0}, "PID gains"=w347, "setpoint"=w354) -> ("output"=w352:dbl)  [unwired: 7 in, 1 out]
          n320 = Multiply(x=w351, y=w352) -> (x*y=w353:dbl)
          n321 = global write "Driver Controller Global.vi" "Output On"(FALSE ("Rumble Controller?")) -> ()
        }
        frame 2 {
          n322 = Multiply(x=0.1, y=w358) -> (x*y=w359:dbl)
        }
      }
    }
  }
  n323 = global write "Drive Train Global.vi" "X Command"(w58) -> ()
